vi "plotall.vi"(11 "Robot Motion Commands":T1) -> ()   [LabVIEW 2016]
uses:
  Robot Motion Commands.ctl
  Motor Commands.ctl
  Robot Drive Mode.ctl
panel:
  out "XY Graph Back Right":cluster{"Array":dbl[], "Array 2":dbl[]}[](graph)
  out "XY Graph Back Left":cluster{"Array":dbl[], "Array 2":dbl[]}[](graph)
  out "XY Graph Front Left":cluster{"Array":dbl[], "Array 2":dbl[]}[](graph)
  out "XY Graph Front Right":cluster{"Array":dbl[], "Array 2":dbl[]}[](graph)
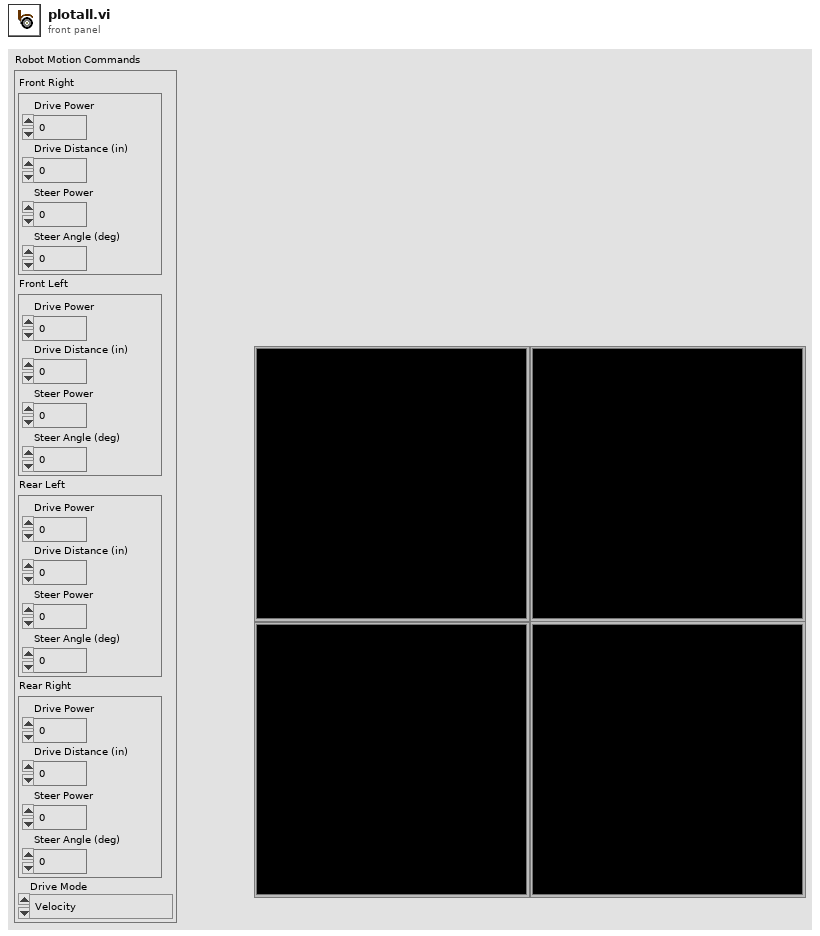
[diagram p1: front panel]
types:
  T1 = typedef "Robot Motion Commands.ctl" = cluster{"Front Right":T2, "Front Left":T2, "Rear Left":T2, "Rear Right":T2, "Drive Mode":T3}
  T2 = typedef "Motor Commands.ctl" = cluster{"Drive Power":dbl, "Drive Distance (in)":dbl, "Steer Power":dbl, "Steer Angle (deg)":dbl}
  T3 = typedef "Robot Drive Mode.ctl" = enum16{"Velocity", "Distance"}
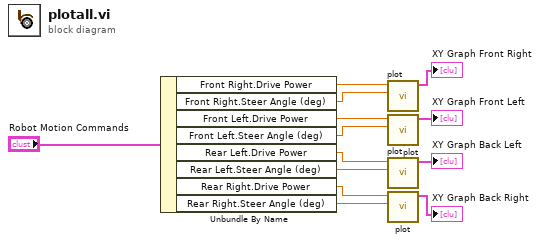
[diagram p0: block diagram]
diagram:
  n1 = Unbundle By Name("Robot Motion Commands") -> ("Front Right.Drive Power"=w8:dbl, "Front Right.Steer Angle (deg)"=w7:dbl, "Front Left.Drive Power"=w6:dbl, "Front Left.Steer Angle (deg)"=w5:dbl, "Rear Left.Drive Power"=w4:dbl, "Rear Left.Steer Angle (deg)"=w3:dbl, "Rear Right.Drive Power"=w2:dbl, "Rear Right.Steer Angle (deg)"=w1:dbl)
  n2 = call "plot.vi"("angle"=w7, "speed"=w8) -> ("XY Graph"=→"XY Graph Front Right":cluster{"Array":dbl[], "Array 2":dbl[]}[])  [unwired: 9 in]
  n3 = call "plot.vi"("angle"=w5, "speed"=w6) -> ("XY Graph"=→"XY Graph Front Left":cluster{"Array":dbl[], "Array 2":dbl[]}[])  [unwired: 9 in]
  n4 = call "plot.vi"("angle"=w3, "speed"=w4) -> ("XY Graph"=→"XY Graph Back Left":cluster{"Array":dbl[], "Array 2":dbl[]}[])  [unwired: 9 in]
  n5 = call "plot.vi"("angle"=w1, "speed"=w2) -> ("XY Graph"=→"XY Graph Back Right":cluster{"Array":dbl[], "Array 2":dbl[]}[])  [unwired: 9 in]
